vi "Rotational Degrees To Ticks.vi"(11 "Rotational Degrees":dbl format="%#_13g") -> (3 "Ticks":dbl format="%#_13g")   [LabVIEW 2016]
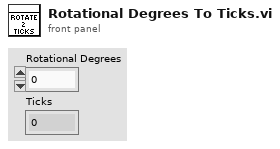
[diagram p1: front panel]
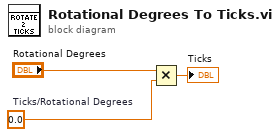
[diagram p0: block diagram]
diagram:
  w2 = 0.0  # Ticks/Rotational Degrees
  n1 = Multiply(x="Rotational Degrees", y=w2) -> (x*y=→"Ticks":dbl)
